vi "save_data_for_flow.vi"(1 "data":i16[][](array[numeric]), 6 "Set pressure":sgl, 7 "Set flow":sgl, 8 "Filename":path, 9 "Sample rate":dbl format="%#_13g", 10 "Sample rate scope":dbl format="%#_13g", 11 "Scope True?":bool=TRUE) -> ()   [LabVIEW 2018]
uses:
  <vilib>/addons/h5labview2/file/H5Fmode.ctl
  <vilib>/addons/h5labview2/base/lib_path.vi
  <vilib>/addons/h5labview2/base/H5Equery.vi
  <vilib>/addons/h5labview2/dataset/H5Dwrite.llb/H5Dwrite.xnode
  <vilib>/addons/h5labview2/attrib/H5Awrite.llb/H5Awrite.xnode
  <vilib>/addons/h5labview2/base/hid_t.ctl
  <vilib>/addons/h5labview2/file/H5F.lvlib
  <vilib>/addons/h5labview2/group/H5G.lvlib
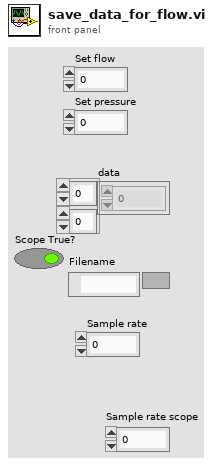
[diagram p1: front panel]
types:
  T1 = typedef "H5F.lvlib/H5Fmode.ctl" = enum16{"read-only", "read-write", "overwrite", "create new", "open or create"}
  T2 = typedef "hid_t.ctl" = i32
  T3 = cluster{"Sample rate":dbl, dbl, "Sample rate scope":dbl}
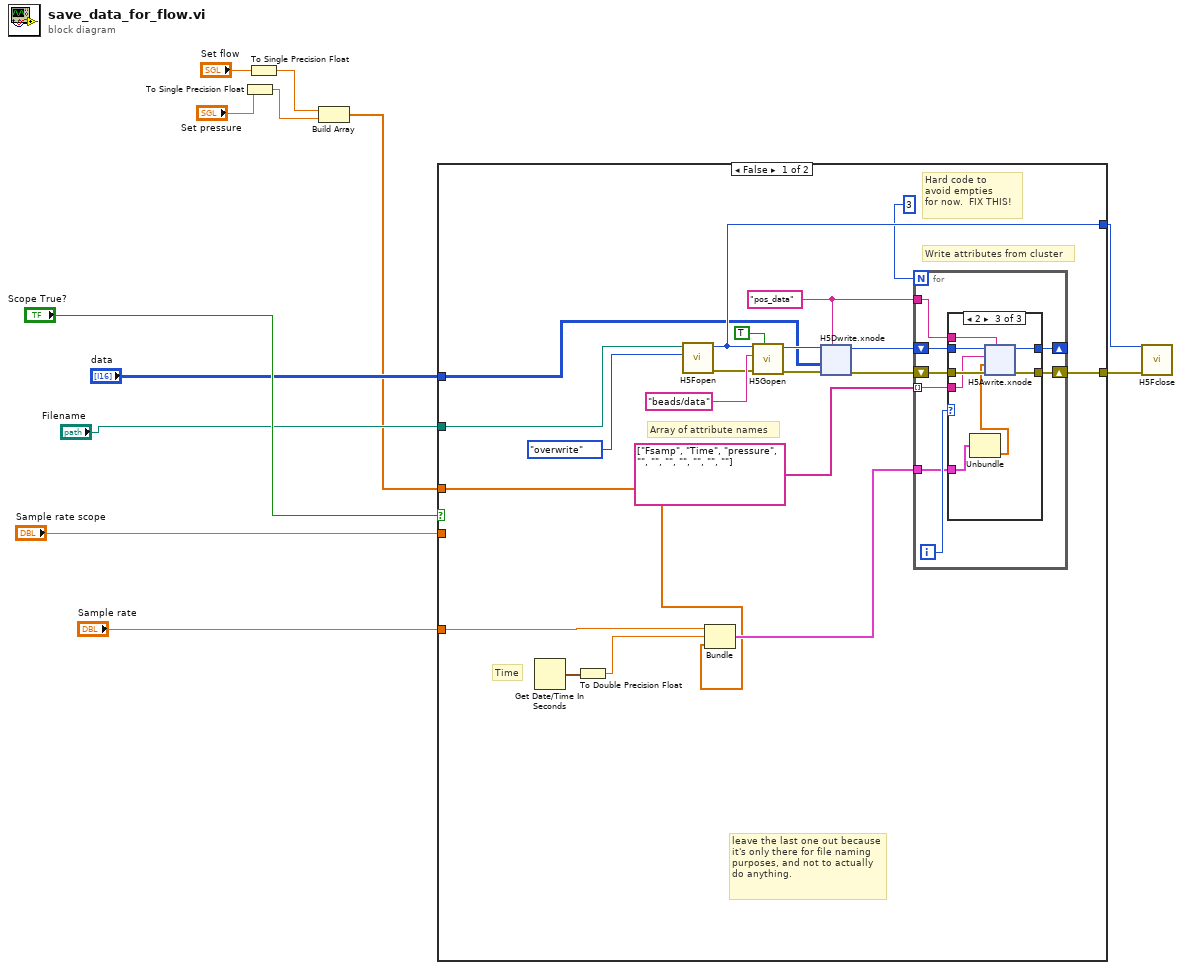
[diagram p0: block diagram]
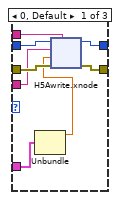
[diagram p2: hidden frame]
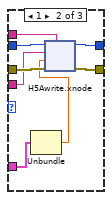
[diagram p3: hidden frame]
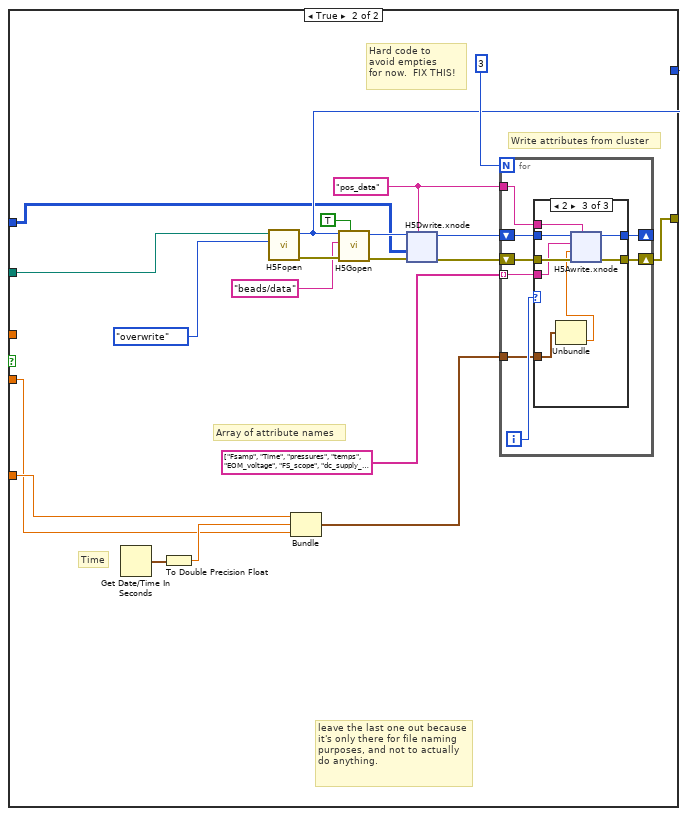
[diagram p4: hidden frame]
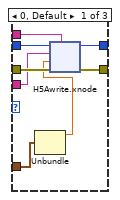
[diagram p5: hidden frame]
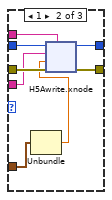
[diagram p6: hidden frame]
diagram:
  n1 = To Single Precision Float(number="Set pressure") -> (single precision float=w3:sgl)
  n2 = To Single Precision Float(number="Set flow") -> (single precision float=w4:sgl)
  n3 = Build Array(w4, w3) -> (w5:sgl[])
  n4 = case shown="False" "Scope True?" {
    tunnel: [w26 w145] -> w12
    tunnel: [w18 w146] -> w11
    tunnel: "Sample rate" -> [w16 w142]
    tunnel: "Filename" -> [w15 w143]
    tunnel: "data" -> [w14 w144]
    tunnel: "Sample rate scope" -> [_ w141]
    tunnel: w5 -> [w13 _]
    frame False {
      w32 = "pos_data" ("dataset name")
      # "leave the last one out because it's only there for file naming purposes, and not to actually do anything."
      # "Hard code to \navoid empties\nfor now.  FIX THIS!"
      # "Time"
      # "Array of attribute names"
      # "Write attributes from cluster"
      n5 = Get Date/Time In Seconds() -> (seconds since 1Jan1904=w28:timestamp)
      n6 = To Double Precision Float(number=w28) -> (double precision float=w21:dbl)
      n7 = call <vilib>:"H5Fopen.vi"("mode (read-only)"=H5Fmode."overwrite", "path"=w15) -> ("error out"=w24:errorcluster, "ref out"=w18:T2)  [unwired: 8 in]
      n8 = Bundle("Sample rate"=w16, w21, w13) -> (w20:cluster{"Sample rate":dbl, dbl, sgl[]})  [unwired: 1 in]
      n9 = call <vilib>:"H5Gopen.vi"("create? (F)"=TRUE, "error in (no error)"=w24, "name"="beads/data", "ref in"=w18) -> ("error out"=w30:errorcluster, "group out"=w19:T2)  [unwired: 6 in]
      n10 = xnode "H5Dwrite.xnode"("dataset name"=w32, "error in (no error)"=w30, "data"=w14, "ref in"=w19) -> ("error out"=w29:errorcluster, "ref out"=w22:i32)  [unwired: 3 in, 1 out]
      n11 = for {
        N: 3 -> [_]
        tunnel: w32 -> [w40]
        shift-right: [w38] -> _
        shift-left: w22 -> [w35]
        shift-right: [w37] -> w26
        shift-left: w29 -> [w39]
        tunnel: string[] ["Fsamp", "Time", "pressure", "", "", "", "", "", "", ""] -> [w36] mode=indexing
        tunnel: w20 -> [w33]
        i -> [w34]
        n12 = case shown="2" w34 {
          tunnel: w40 -> [w48 w75 w102]
          tunnel: w39 -> [w47 w74 w101]
          tunnel: [w46 w73 w100] -> w38
          tunnel: [w45 w72 w99] -> w37
          tunnel: w36 -> [w44 w71 w98]
          tunnel: w35 -> [w43 w70 w97]
          tunnel: w33 -> [w42 w69 w96]
          frame 0, Default {
            n13 = Unbundle(w42) -> ("Sample rate"=w41:dbl)  [unwired: 2 out]
            n14 = xnode "H5Awrite.xnode"("object name"=w48, "error in (no error)"=w47, "data"=w41, "attrib name"=w44, "ref in"=w43) -> ("error out"=w45:errorcluster, "ref out"=w46:T2)  [unwired: 2 in, 1 out]
          }
          frame 1 {
            n15 = Unbundle(w69) -> (w68:dbl)  [unwired: 2 out]
            n16 = xnode "H5Awrite.xnode"("object name"=w75, "error in (no error)"=w74, "data"=w68, "attrib name"=w71, "ref in"=w70) -> ("error out"=w72:errorcluster, "ref out"=w73:T2)  [unwired: 2 in, 1 out]
          }
          frame 2 {
            n17 = Unbundle(w96) -> (w95:sgl[])  [unwired: 2 out]
            n18 = xnode "H5Awrite.xnode"("object name"=w102, "error in (no error)"=w101, "data"=w95, "attrib name"=w98, "ref in"=w97) -> ("error out"=w99:errorcluster, "ref out"=w100:T2)  [unwired: 2 in, 1 out]
          }
        }
      }
    }
    frame True {
      w147 = "pos_data" ("dataset name")
      # "leave the last one out because it's only there for file naming purposes, and not to actually do anything."
      # "Hard code to \navoid empties\nfor now.  FIX THIS!"
      # "Time"
      # "Array of attribute names"
      # "Write attributes from cluster"
      n19 = Get Date/Time In Seconds() -> (seconds since 1Jan1904=w151:timestamp)
      n20 = To Double Precision Float(number=w151) -> (double precision float=w157:dbl)
      n21 = call <vilib>:"H5Fopen.vi"("mode (read-only)"=H5Fmode."overwrite", "path"=w143) -> ("error out"=w154:errorcluster, "ref out"=w146:T2)  [unwired: 8 in]
      n22 = Bundle("Sample rate"=w142, w157, "Sample rate scope"=w141) -> (w158:T3)  [unwired: 1 in]
      n23 = call <vilib>:"H5Gopen.vi"("create? (F)"=TRUE, "error in (no error)"=w154, "name"="beads/data", "ref in"=w146) -> ("error out"=w149:errorcluster, "group out"=w159:T2)  [unwired: 6 in]
      n24 = xnode "H5Dwrite.xnode"("dataset name"=w147, "error in (no error)"=w149, "data"=w144, "ref in"=w159) -> ("error out"=w150:errorcluster, "ref out"=w156:i32)  [unwired: 3 in, 1 out]
      n25 = for {
        N: 3 -> [_]
        tunnel: w147 -> [w168]
        shift-right: [w166] -> _
        shift-left: w156 -> [w163]
        shift-right: [w165] -> w145
        shift-left: w150 -> [w167]
        tunnel: string[] ["Fsamp", "Time", "pressures", "temps", "EOM_voltage", "FS_scope", "dc_supply_settings", "electrode_dc_vals", "stage_settings"] -> [w164] mode=indexing
        tunnel: w158 -> [w161]
        i -> [w162]
        n26 = case shown="2" w162 {
          tunnel: w168 -> [w176 w203 w230]
          tunnel: w167 -> [w175 w202 w229]
          tunnel: [w174 w201 w228] -> w166
          tunnel: [w173 w200 w227] -> w165
          tunnel: w164 -> [w172 w199 w226]
          tunnel: w163 -> [w171 w198 w225]
          tunnel: w161 -> [w170 w197 w224]
          frame 0, Default {
            n27 = Unbundle(w170) -> ("Sample rate"=w169:dbl)  [unwired: 2 out]
            n28 = xnode "H5Awrite.xnode"("object name"=w176, "error in (no error)"=w175, "data"=w169, "attrib name"=w172, "ref in"=w171) -> ("error out"=w173:errorcluster, "ref out"=w174:T2)  [unwired: 2 in, 1 out]
          }
          frame 1 {
            n29 = Unbundle(w197) -> (w196:dbl)  [unwired: 2 out]
            n30 = xnode "H5Awrite.xnode"("object name"=w203, "error in (no error)"=w202, "data"=w196, "attrib name"=w199, "ref in"=w198) -> ("error out"=w200:errorcluster, "ref out"=w201:T2)  [unwired: 2 in, 1 out]
          }
          frame 2 {
            n31 = Unbundle(w224) -> ("Sample rate scope"=w223:dbl)  [unwired: 2 out]
            n32 = xnode "H5Awrite.xnode"("object name"=w230, "error in (no error)"=w229, "data"=w223, "attrib name"=w226, "ref in"=w225) -> ("error out"=w227:errorcluster, "ref out"=w228:T2)  [unwired: 2 in, 1 out]
          }
        }
      }
    }
  }
  n33 = call <vilib>:"H5Fclose.vi"("error in (no error)"=w12, "ref"=w11) -> ()  [unwired: 9 in, 1 out]
